vi "smooth.vi"(11 "Array":i32[](array[numeric])) -> (3 "Array 2":i32[](array[numeric]))   [LabVIEW 2012]
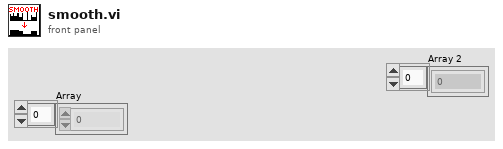
[diagram p1: front panel]
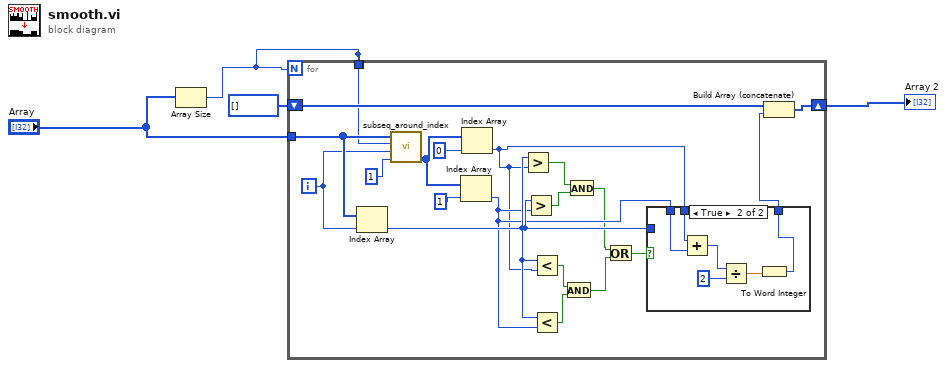
[diagram p0: block diagram]
diagram:
  n1 = Array Size(array="Array") -> (size(s)=w2:i32)
  n2 = for {
    N: w2 -> [_]
    tunnel: "Array" -> [w22]
    shift-right: [w24] -> w3
    shift-left: i8[] [] -> [w20]
    tunnel: w2 -> [_]
    tunnel: w2 -> [w13]
    i -> [w21]
    n3 = Index Array(array=w22, index=w21) -> (element=w12:i32)
    n4 = call "subseq_around_index.vi"("length around index 2"=1, "index 2"=w21, "array length 2"=w13, "Array 3"=w22) -> ("Array 2"=w19:i32[])  [unwired: 7 in]
    n5 = Index Array(array=w19, index=1 ("length around index 2")) -> (element=w11:i32)
    n6 = Index Array(array=w19, index=0 ("length around index 2")) -> (element=w10:i32)
    n7 = Greater?(x=w12, y=w10) -> (0:w16:bool)
    n8 = Greater?(x=w12, y=w11) -> (0:w15:bool)
    n9 = Less?(x=w12, y=w10) -> (x < y?=w9:bool)
    n10 = Less?(x=w12, y=w11) -> (x < y?=w8:bool)
    n11 = And(x=w9, y=w8) -> (x .and. y?=w5:bool)
    n12 = And(x=w16, y=w15) -> (x .and. y?=w6:bool)
    n13 = Or(x=w6, y=w5) -> (x .or. y?=w7:bool)
    n14 = case shown="True" w7 {
      tunnel: w12 -> [w25 _]
      tunnel: w10 -> [_ w30]
      tunnel: w11 -> [_ w29]
      tunnel: [w25 w27] -> w14
      frame False {
      }
      frame True {
        n15 = Add(x=w30, y=w29) -> (x+y=w31:i32)
        n16 = Divide(x=w31, y=2) -> (x/y=w28:dbl)
        n17 = To Word Integer(number=w28) -> (16bit integer=w27:i16)
      }
    }
    n18 = Build Array (concatenate)(w20, w14) -> (w24:i32[])
  }
  "Array 2" <- w3
